vi "Parse DOSCAR.vi"(8 "error in (no error)":errorcluster, 10 "Only total DOS":bool=TRUE, 11 "Path":path=path "C:/Users/Chris B/Documents/Ab Initio/Vasp Calcs 1/Batch2_20130416") -> (0 "error out":errorcluster, 1 "Atomic-decomposed DOS":T2(array[cluster]), 2 "Total DOS":T1, 3 "DOS Summary":T3)   [LabVIEW 2010]
uses:
  <vilib>/Utility/file.llb/Read From Spreadsheet File (string).vi
  <vilib>/Analysis/8numeric.llb/1D Numeric Integration.vi
  <vilib>/Analysis/NI_AALBase.lvlib
  <vilib>/Analysis/NI_AALPro.lvlib
panel:
  out "Density of Condution Band":dbl
  out "Density of Valence Band":dbl
  out "# States":dbl
  out "Fermi Level (eV)":dbl
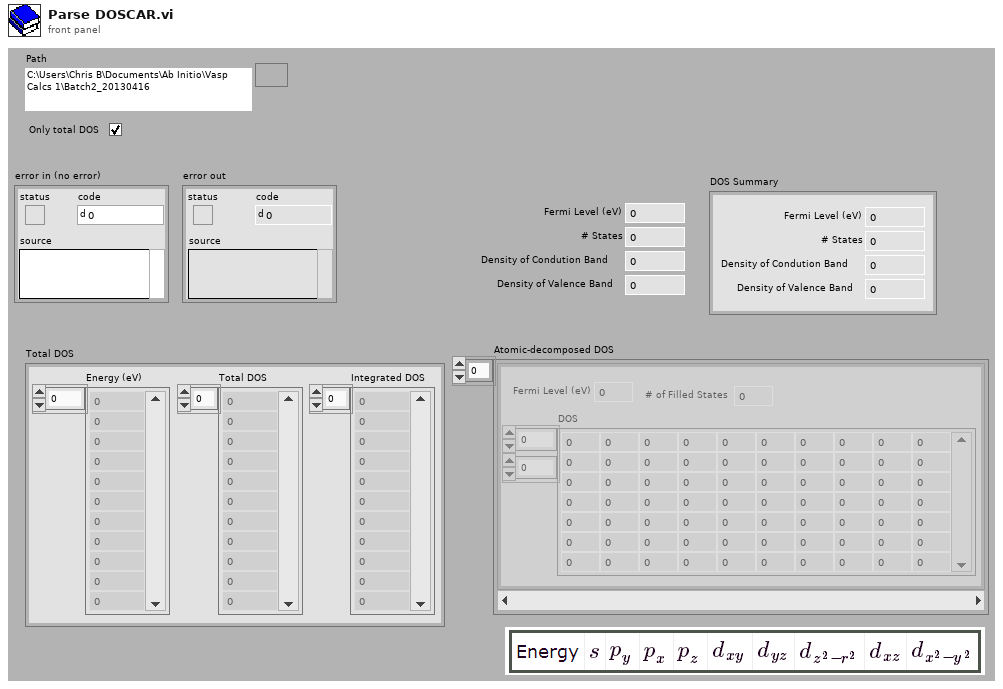
[diagram p1: front panel]
types:
  T1 = cluster{"Energy (eV)":dbl[], "Total DOS":dbl[], "Integrated DOS":dbl[]}
  T2 = cluster{"Fermi Level (eV)":dbl, "# of Filled States":dbl, "DOS":dbl[][]}[]
  T3 = cluster{"Fermi Level (eV)":dbl, "# States":dbl, "Density of Valence Band":dbl, "Density of Condution Band":dbl}
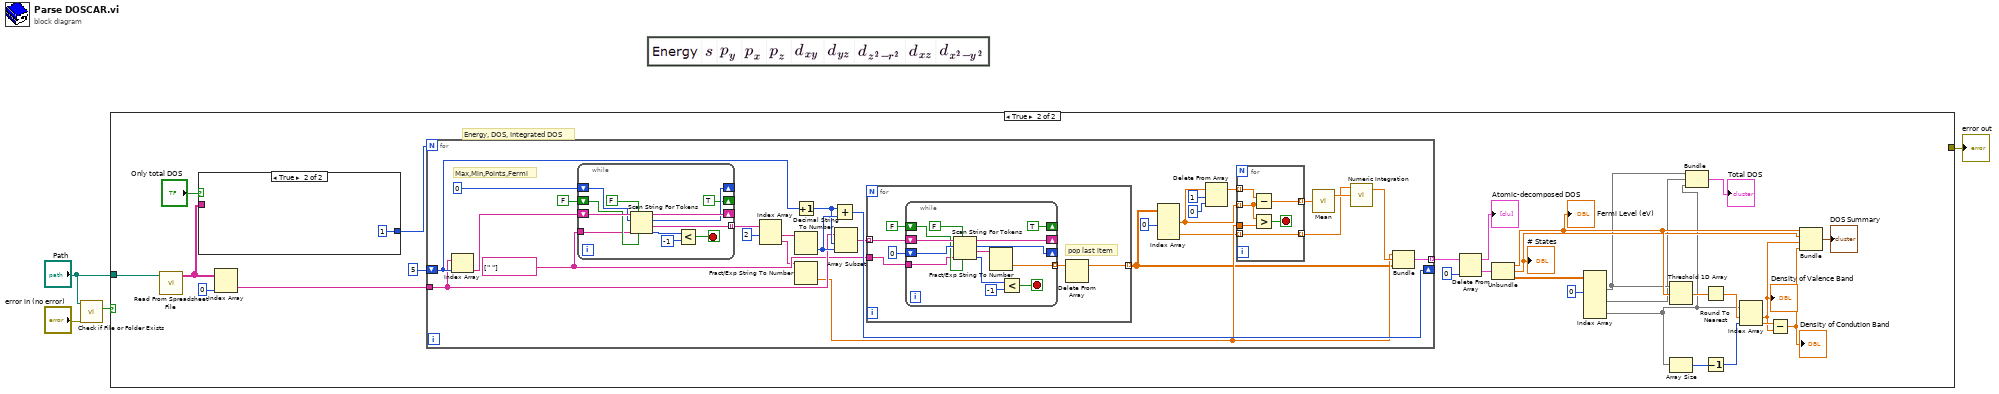
[diagram p0: block diagram]
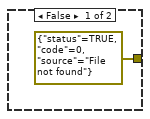
[diagram p2: hidden frame]
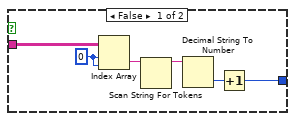
[diagram p3: hidden frame]
diagram:
  n1 = call <vilib>:"Check if File or Folder Exists.vi"("error in (no error)"="error in (no error)", "path"="Path") -> ("file or folder exists?"=w3:bool)  [unwired: 7 in, 2 out]
  n2 = case shown="True" w3 {
    tunnel: "Path" -> [_ w26]
    tunnel: [errorcluster {"status"=TRUE, "code"=0, "source"="File not found"} ("error out") _] -> w2
    frame False {
    }
    frame True {
      # "Energy, DOS, Integrated DOS"
      n3 = call-poly <vilib>:"Read From Spreadsheet File.vi"("file path (dialog if empty)"=w26) -> ("all rows"=w30:string[][])  [unwired: 6 in, 4 out]
      n4 = case shown="True" "Only total DOS" {
        tunnel: [w36 1] -> w31
        tunnel: w30 -> [w35 _]
        frame False {
          w38 = 0 ("index (row)")
          n5 = Index Array(array=w35, index (row)=w38, index (col)=w38) -> (element=w34:string)
          n6 = Scan String For Tokens(9:w34) -> (3:w33:string)  [unwired: 5 in, 3 out]
          n7 = Decimal String To Number(string=w33) -> (number=w37:i32)  [unwired: 2 in, 1 out]
          n8 = Increment(x=w37) -> (x+1=w36:i32)
        }
        frame True {
        }
      }
      n9 = Index Array(array=w30, index (col)=0 ("disabled index (col)")) -> (element=w28:string[])  [unwired: 1 in]
      n10 = for {
        N: w31 -> [_]
        shift-right: [w61] -> _
        shift-left: 5 ("disabled index (col)") -> [w63]
        tunnel: [w64] -> w15 mode=indexing
        tunnel: w28 -> [w56]
        w54 = string[] [" "] ("delimiters (\\s,\\t,\\r,\\n)")
        # "Max,Min,Points,Fermi"
        n11 = Index Array(array=w56, index=w63) -> (element=w59:string)
        n12 = while {
          shift-right: [w101] -> _
          shift-left: w59 -> [w102]
          tunnel: [w100] -> w57 mode=indexing
          shift-right: [w99] -> _
          shift-left: 0 ("offset past token") -> [w98]
          shift-right: [TRUE ("allow empty tokens? (F)")] -> _
          shift-left: FALSE ("allow empty tokens? (F)") -> [w94]
          tunnel: w54 -> [w92]
          stop <- w95 stop-if-true
          n13 = Scan String For Tokens(4:w94, 5:FALSE ("allow empty tokens? (F)"), 6:w92, 8:w98, 9:w102) -> (0:w97:i32, 1:w100:string, 2:w99:i32, 3:w101:string)  [unwired: 1 in]
          n14 = Less?(x=w97, y=-1) -> (x < y?=w95:bool)
        }
        n15 = Index Array(array=w57, index #1=2 ("index")) -> (element #1=w65:string, element #2=w52:string)  [unwired: 1 in]
        n16 = Increment(x=w63) -> (x+1=w60:i32)
        n17 = Decimal String To Number(string=w65) -> (number=w62:i32)  [unwired: 2 in, 1 out]
        n18 = Fract/Exp String To Number(string=w52) -> (number=w43:dbl)  [unwired: 3 in, 1 out]
        n19 = Add(x=w60, y=w62) -> (x+y=w61:i32)
        n20 = Array Subset(array=w56, index=w60, length=w62) -> (w55:string[])
        n21 = for {
          tunnel: w55 -> [w78] mode=indexing
          tunnel: w54 -> [w77]
          tunnel: [w73] -> w40 mode=indexing
          # "pop last item"
          n22 = while {
            shift-right: [w89] -> _
            shift-left: w78 -> [w90]
            shift-right: [w88] -> _
            shift-left: 0 ("offset past token") -> [w87]
            shift-right: [TRUE ("allow empty tokens? (F)")] -> _
            shift-left: FALSE ("allow empty tokens? (F)") -> [w83]
            tunnel: w77 -> [w81]
            tunnel: [w79] -> w74 mode=indexing
            stop <- w84 stop-if-true
            n23 = Scan String For Tokens(4:w83, 5:FALSE ("allow empty tokens? (F)"), 6:w81, 8:w87, 9:w90) -> (0:w86:i32, 1:w80:string, 2:w88:i32, 3:w89:string)  [unwired: 1 in]
            n24 = Fract/Exp String To Number(string=w80) -> (number=w79:dbl)  [unwired: 3 in, 1 out]
            n25 = Less?(x=w86, y=-1) -> (x < y?=w84:bool)
          }
          n26 = Delete From Array(array=w74) -> (array with subset deleted=w73:dbl[])  [unwired: 2 in, 1 out]
        }
        n27 = Index Array(array=w40, index (col) #1=0 ("disabled index (col)")) -> (element #1=w50:dbl[], element #2=w41:dbl[])  [unwired: 3 in]
        n28 = Delete From Array(array=w50, length=1, index=0) -> (array with subset deleted=w48:dbl[])  [unwired: 1 out]
        n29 = for {
          tunnel: w50 -> [w70] mode=indexing
          tunnel: w48 -> [w72] mode=indexing
          tunnel: [w71] -> w46 mode=indexing
          tunnel: w43 -> [w69]
          tunnel: [w67] -> w42 mode=indexing
          tunnel: w41 -> [w67] mode=indexing
          stop <- w68 stop-if-true
          n30 = Subtract(x=w72, y=w70) -> (x-y=w71:dbl)
          n31 = Greater?(x=w70, y=w69) -> (0:w68:bool)
        }
        n32 = call <vilib>:"Mean.vi"("X"=w46) -> ("mean"=w47:dbl)  [unwired: 1 out]
        n33 = call-poly <vilib>:"Numeric Integration.vi"("dt"=w47, "Input Array"=w42) -> ("result"=w45:dbl)  [unwired: 1 in, 1 out]
        n34 = Bundle(w43, "result"=w45, w40) -> (w64:cluster{dbl, "result":dbl, dbl[][]})  [unwired: 1 in]
      }
      n35 = Delete From Array(array=w15, index=0) -> (deleted portion=w11:cluster{dbl, "result":dbl, dbl[][]}, array with subset deleted=→"Atomic-decomposed DOS":cluster{dbl, "result":dbl, dbl[][]}[])  [unwired: 1 in]
      n36 = Unbundle(w11) -> (w22:dbl, "result"=w21:dbl, w10:dbl[][])
      "Fermi Level (eV)" <- w22
      "# States" <- w21
      n37 = Index Array(array=w10, index (col) #1=0 ("disabled index (col)")) -> (element #1=w9:dbl[], element #2=w8:dbl[], element #3=w7:dbl[])  [unwired: 5 in]
      n38 = Threshold 1D Array(2:w22, 3:w9) -> (0:w17:dbl)  [unwired: 1 in]
      n39 = Array Size(array=w7) -> (size(s)=w25:i32)
      n40 = Bundle(w9, w8, w7) -> (→"Total DOS":cluster{dbl[], dbl[], dbl[]})  [unwired: 1 in]
      n41 = Round To Nearest(number=w17) -> (nearest integer value=w16:dbl)
      n42 = Decrement(x=w25) -> (x-1=w24:i32)
      n43 = Index Array(array=w7, index #1=w16, index #2=w24) -> (element #1=w20:dbl, element #2=w23:dbl)
      "Density of Valence Band" <- w20
      n44 = Subtract(x=w23, y=w20) -> (x-y=w19:dbl)
      "Density of Condution Band" <- w19
      n45 = Bundle(w22, "result"=w21, w20, w19) -> (→"DOS Summary":cluster{dbl, "result":dbl, dbl, dbl})  [unwired: 1 in]
    }
  }
  "error out" <- w2
